vi "超声波对正(子VI).vi"(9 "LFT":dbl=70000.0 format="%#_13g", 10 "FWD":dbl=100000.0 format="%#_13g", 11 "超声波":dbl[](array[numeric])) -> (3 "数组输出":dbl[](array[numeric]))   [LabVIEW 2017]
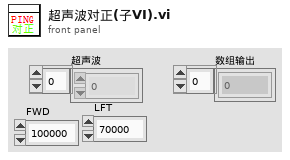
[diagram p1: front panel]
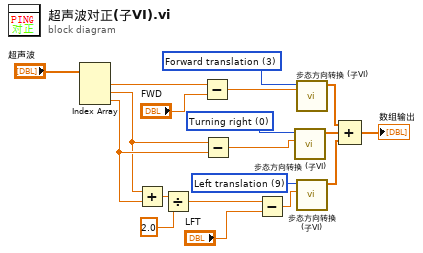
[diagram p0: block diagram]
diagram:
  w17 = i8 9 items=["Stop"=-1, "Right translation"=6, "Back translation"=12, "Turning right"=0, "Turning left"=15, "Forward translation"=3, "Left translation"=9, "Gyro rotating"=16] ("Gait")
  w6 = i8 0 items=["Stop"=-1, "Right translation"=6, "Back translation"=12, "Turning right"=0, "Turning left"=15, "Forward translation"=3, "Left translation"=9, "Gyro rotating"=16] ("Gait")
  w5 = i8 3 items=["Stop"=-1, "Right translation"=6, "Back translation"=12, "Turning right"=0, "Turning left"=15, "Forward translation"=3, "Left translation"=9, "Gyro rotating"=16] ("Gait")
  n1 = Index Array(array="超声波") -> (element #1=w2:dbl, element #2=w11:dbl, element #3=w12:dbl)  [unwired: 3 in]
  n2 = Add(x=w11, y=w12) -> (x+y=w13:dbl)
  n3 = Divide(x=w13, y=2.0) -> (x/y=w15:dbl)
  n4 = Subtract(x=w2, y="FWD") -> (x-y=w4:dbl)
  n5 = Subtract(x=w11, y=w12) -> (x-y=w7:dbl)
  n6 = Subtract(x=w15, y="LFT") -> (x-y=w18:dbl)
  n7 = call "步态方向转换 (子VI).vi"("速度"=w7, "Gait"=w6) -> ("输出"=w9:dbl[])  [unwired: 9 in]
  n8 = call "步态方向转换 (子VI).vi"("速度"=w4, "Gait"=w5) -> ("输出"=w8:dbl[])  [unwired: 9 in]
  n9 = call "步态方向转换 (子VI).vi"("速度"=w18, "Gait"=w17) -> ("输出"=w19:dbl[])  [unwired: 9 in]
  n10 = Compound Arithmetic op=ADD(w8, w9, w19) -> (→"数组输出":dbl[])
